vi "re_DataLog Mirror Module.vi"(5 "LuaVIEW reference":T1, 7 "function index":i32) -> (15 "error out":errorcluster)   [LabVIEW 2012]
doc: "Module required by the \"mirroring\" runlevel if mirrored databases have been configured. It assists with the mirroring of a remote logging database. It is reentrant so that it can be instantiated multiple times, once for each database being mirrored."
uses:
  luaview/typedefs/t_LuaVIEW Reference.ctl
  typedefs/clusters/t_DataLog Tag Config.ctl
  typedefs/t_DataLog Temporal Types.ctl
  typedefs/t_DataLog Value Types.ctl
  typedefs/t_DataLog Numerical Format.ctl
  typedefs/t_DataLog Logging Algorithms.ctl
  typedefs/t_DataLog Mirror State Methods.ctl
  clientsrv/served/ClientSrv Server Access_srv.ctl
  clientsrv/typedefs/t_ClientSrv Server Access Methods.ctl
  clientsrv/typedefs/t_ClientSrv Access Levels.ctl
  served/DataLog Mirror_srv.ctl
  served/DataLog Database Infos_srv.ctl
  typedefs/t_DataLog Tag Info List Methods.ctl
  typedefs/t_DataLog Databases Methods.ctl
  luaview/subvis/private/LuaVIEW Pull (flat data).vi
  luaview/subvis/private/LuaVIEW Pull (refnum).vi
  luaview/subvis/private/LuaVIEW Pull (string).vi
  luaview/subvis/private/LuaVIEW Push (string).vi
  luaview/subvis/private/re_LuaVIEW Push (flat data).vi
  luaview/subvis/private/LuaVIEW Push (I32).vi
  luaview/subvis/private/LuaVIEW Pull (I32).vi
  luaview/subvis/private/LuaVIEW Push (boolean).vi
  luaview/subvis/private/LuaVIEW Push (number).vi
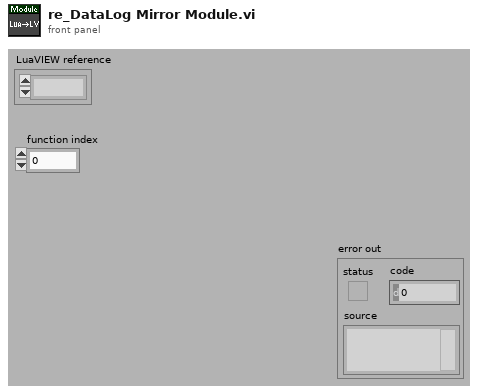
[diagram p1: front panel]
types:
  T1 = typedef "t_LuaVIEW Reference.ctl" = refnum<k1>
  T2 = typedef "t_DataLog Tag Config.ctl" = cluster{"name":string, "unit":string, "temporal":T3, "value":T4, "index":i32, "capacity":i32, "is meta?":bool, "mincapacity":i32, "deadband":dbl, "limit delay":dbl, "format":T5, "precision":u8, "undefine":bool, "update":bool, "update period":u16, "expression":string, "description":string, "logging algorithm":T6, "logging parameters":dbl[]}
  T3 = typedef "t_DataLog Temporal Types.ctl" = enum16{"set&hold", "sample", "event"}
  T4 = typedef "t_DataLog Value Types.ctl" = enum16{"number", "string"}
  T5 = typedef "t_DataLog Numerical Format.ctl" = enum8{"fractional", "exponential", "engineering"}
  T6 = typedef "t_DataLog Logging Algorithms.ctl" = enum16{"nothing", "changes", "everything", "every Nth", "time threshold", "value threshold + prior", "t or v threshold", "t or v threshold + prior"}
  T7 = enum32{"initialize", "str:server=connect()", "num:changecount,tab:taglist=get_list(num:changecount)", "create_empty(tab:config)", "bool:mirrored=mirror_config(tab:remote_config)", "bool:mirrored=mirror_subsets()", "num:mirrored_values=mirror_tag(str:tag)", "str:name=localdb()", "str:name=remotedb()", "disconnect()"}
  T8 = typedef "t_DataLog Mirror State Methods.ctl" = enum16{"add db", "check db", "set", "get", "unset", "clear"}
  T9 = typedef "ClientSrv Server Access_srv.ctl" = refnum<vi>
  T10 = typedef "DataLog Database Infos_srv.ctl" = refnum<vi>
  T11 = typedef "DataLog Mirror_srv.ctl" = refnum<vi>
  T12 = typedef "t_ClientSrv Access Levels.ctl" = enum16{"observer", "operator", "local"}
  T13 = typedef "t_ClientSrv Server Access Methods.ctl" = enum16{"validate access", "test access", "release access", "get name"}
  T14 = typedef "t_DataLog Tag Info List Methods.ctl" = enum16{"initialize", "create", "create empty", "rename", "delete", "test tag", "get", "get by name", "get default", "get list", "get path", "get subsets", "set subsets", "set config", "set capacity", "#tags", "go live", "set unlocked", "set mirrored"}
  T15 = typedef "t_DataLog Databases Methods.ctl" = enum16{"initialize", "get ref", "get names", "cleanup"}
  T16 = cluster{"localdb":string, "remotedb":string, "machine":string, "port":u32, "password":string}
  T17 = enum32{"invalid app kind", "Development System", "Run Time System", "Student Edition", "Embedded LabVIEW", "Evaluation", "Custom"}
  T18 = typedef "t_DataLog Database Info Pane.ctl" = refnum<vi>
  T19 = typedef "et_DataLog Meta Tag Specifier.ctl" = enum32{"warn_lo", "warn_hi", "A_lo", "A_hi", "B_lo", "B_hi", "C_lo", "C_hi", "D_lo", "D_hi", "E_lo", "E_hi", "F_lo", "F_hi", "G_lo", "G_hi", "H_lo", "H_hi", "I_lo", "I_hi", "J_lo", "J_hi", "K_lo", "K_hi", "L_lo", "L_hi", "M_lo", "M_hi", "N_lo", "N_hi", "min", "max", "not a meta"}
  T20 = typedef "t_DataLog Tag Subset.ctl" = cluster{"name":string, "tags":string[]}
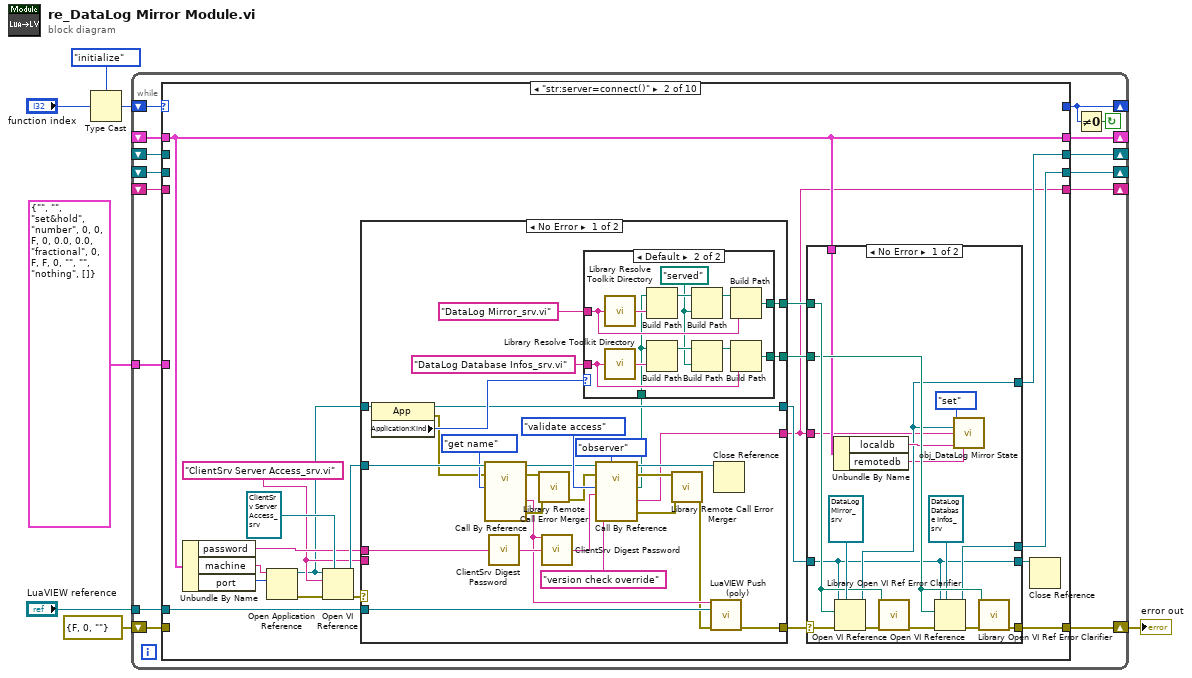
[diagram p0: block diagram]
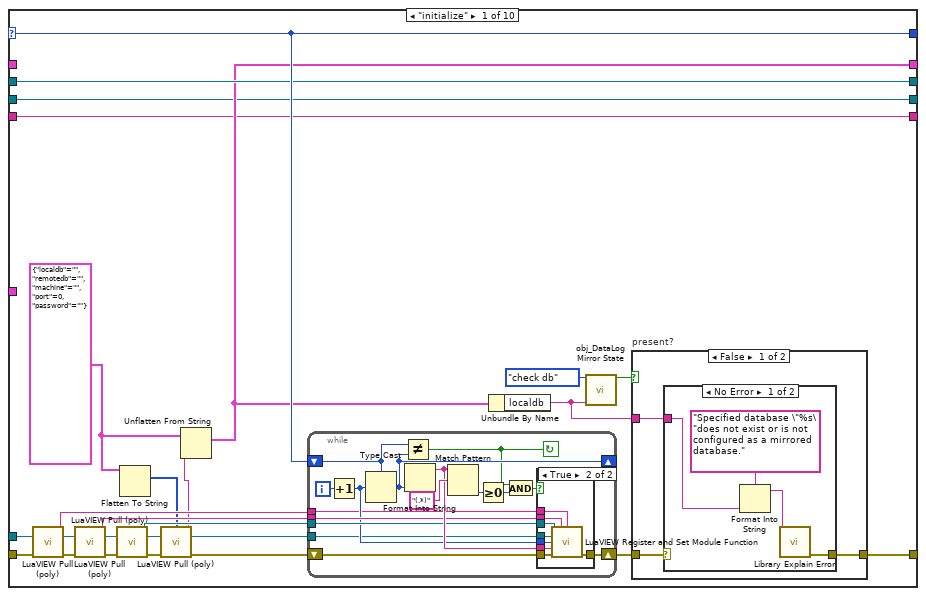
[diagram p2: hidden frame]
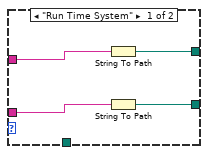
[diagram p7: hidden frame]
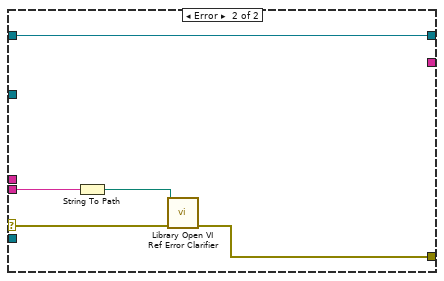
[diagram p8: hidden frame]
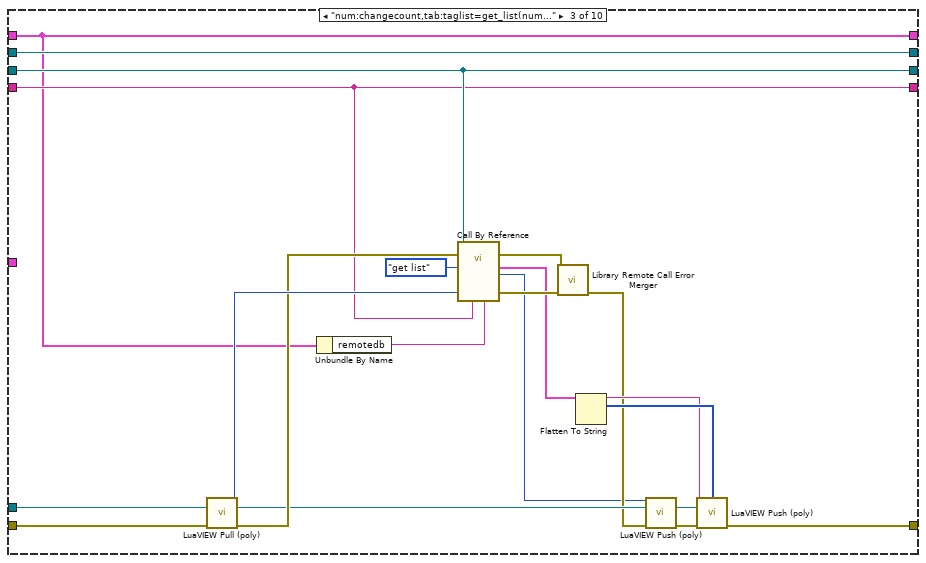
[diagram p9: hidden frame]
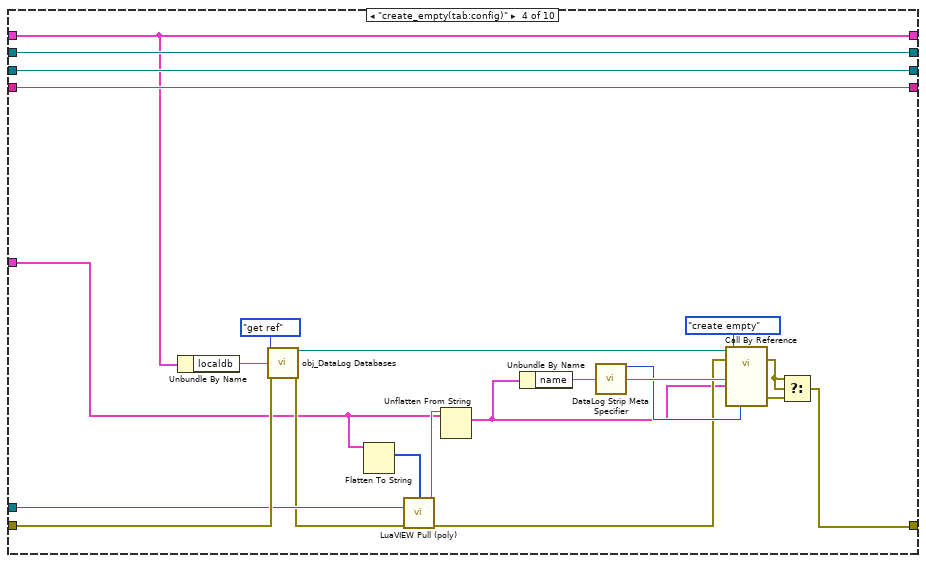
[diagram p10: hidden frame]
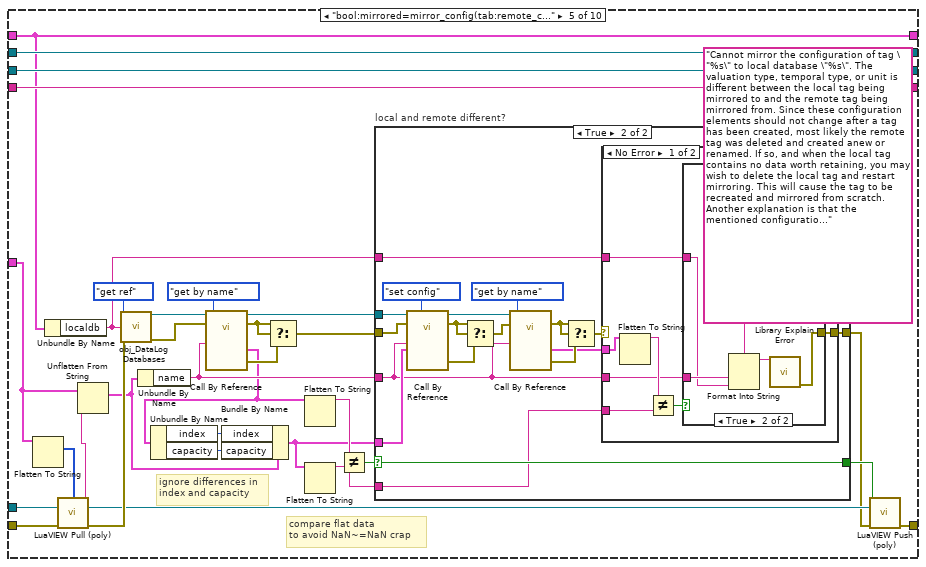
[diagram p11: hidden frame]
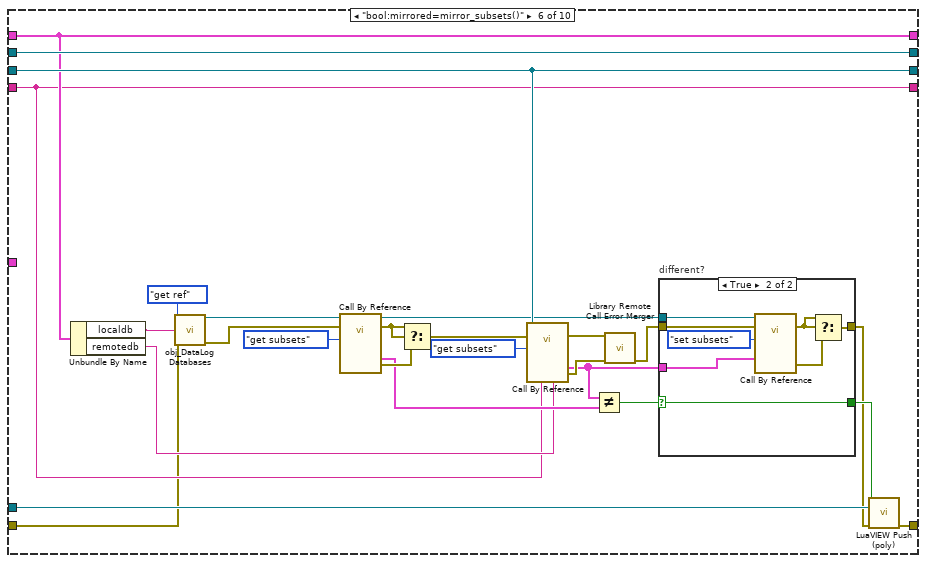
[diagram p15: hidden frame]
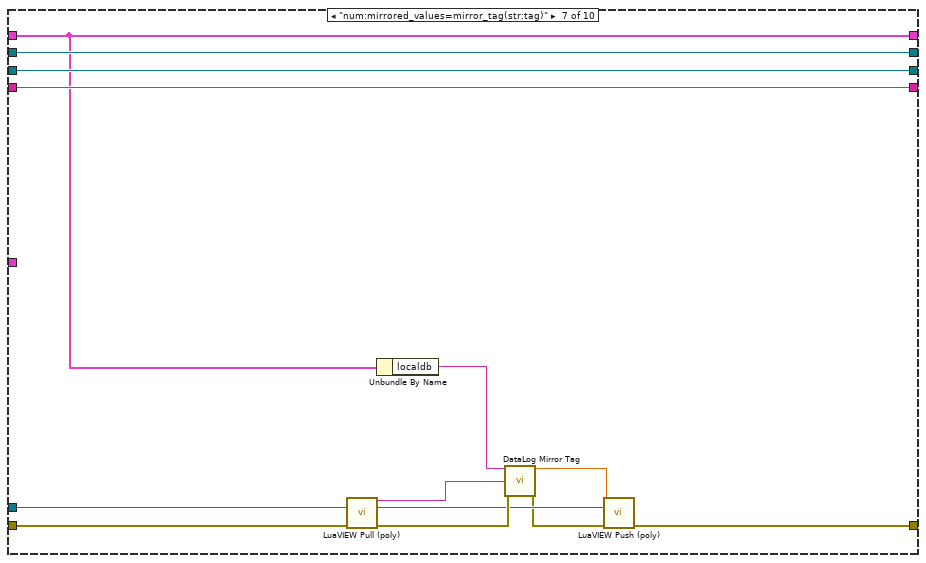
[diagram p17: hidden frame]
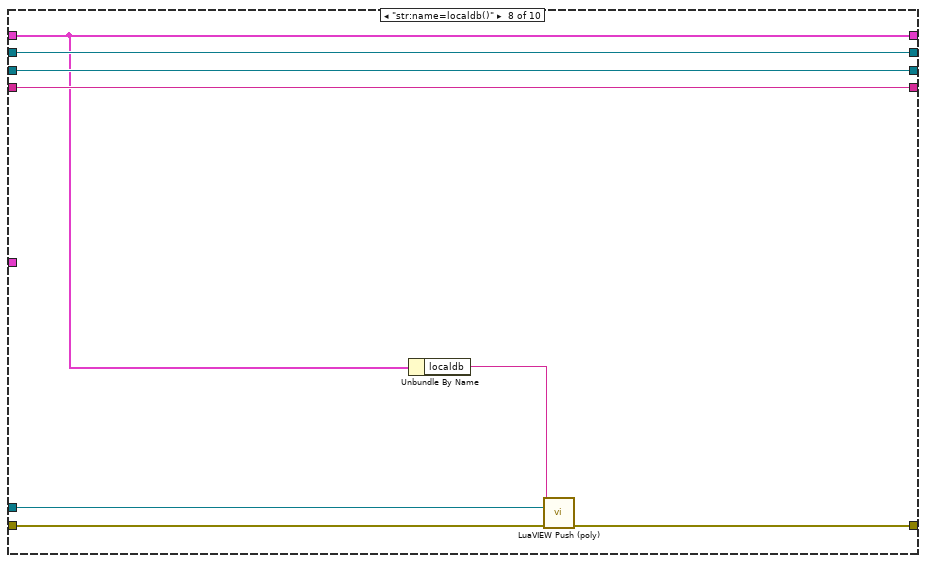
[diagram p18: hidden frame]
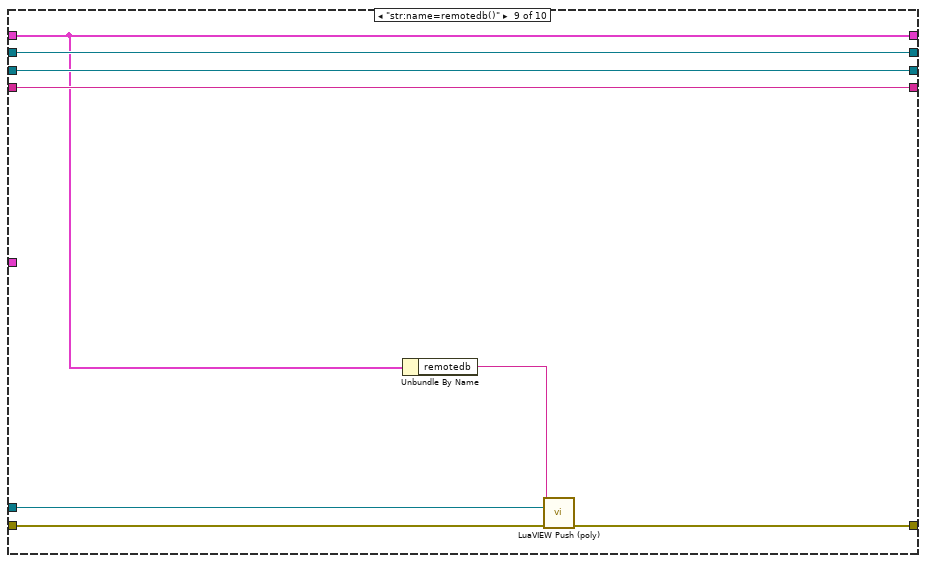
[diagram p19: hidden frame]
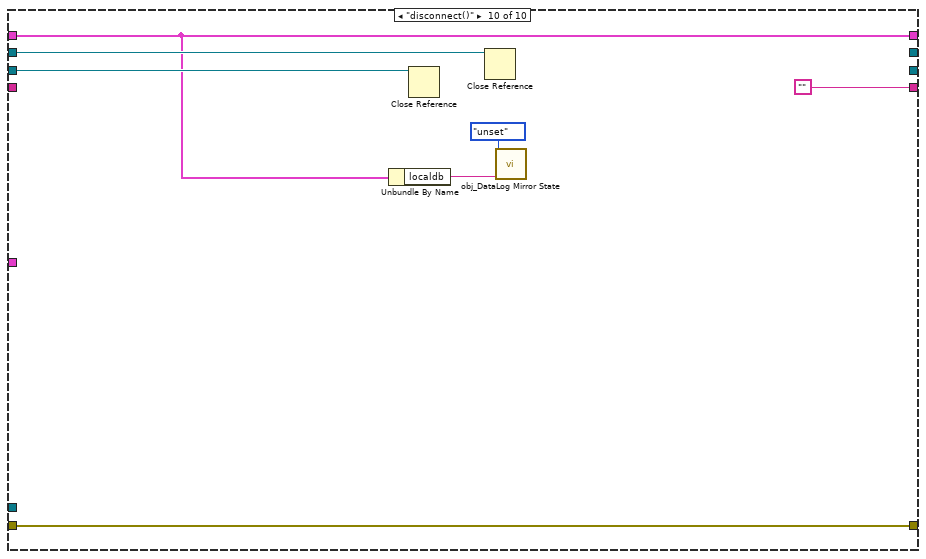
[diagram p20: hidden frame]
diagram:
  n1 = Type Cast(type=T7."initialize" ("cases"), x="function index") -> (*(type *) &x=w6:T7)
  n2 = while {
    shift-right: [w18] -> _
    shift-left: w6 -> [w22]
    shift-right: [w21] -> w7
    shift-left: errorcluster {"status"=FALSE, "code"=0, "source"=""} ("error out") -> [w20]
    tunnel: "LuaVIEW reference" -> [w19]
    shift-right: [w16] -> _
    shift-left: _ -> [w15]
    shift-right: [w14] -> _
    shift-left: _ -> [w13]
    shift-right: [w12] -> _
    shift-left: _ -> [w11]
    shift-right: [w10] -> _
    shift-left: _ -> [w9]
    tunnel: T2 {"name"="", "unit"="", "temporal"=enum."set&hold", "value"=enum."number", "index"=0, "capacity"=0, "is meta?"=FALSE, "mincapacity"=0, "deadband"=0.0, "limit delay"=0.0, "format"=enum."fractional", "precision"=0, "undefine"=FALSE, "update"=FALSE, "update period"=0, "expression"="", "description"="", "logging algorithm"=enum."nothing", "logging parameters"=[]} ("tag config") -> [w8]
    stop <- w17 continue-if-true
    n3 = case shown="\"str:server=connect()\"" w22 {
      selector: w22 -> [w39 _ _ _ _ _ _ _ _ _]
      tunnel: [w39 _ _ _ _ _ _ _ _ _] -> w18
      tunnel: w19 -> [w41 w95 w188 w197 w240 w305 w321 w331 w339 _]
      tunnel: [w27 w93 w183 w203 w226 w304 w317 w330 w338 w351] -> w21
      tunnel: w20 -> [w40 _ w189 w198 w241 w281 w324 w332 w340 w351]
      tunnel: [w31 w85 w173 w202 w243 w298 w325 w333 w341 w347] -> w16
      tunnel: w15 -> [_ w85 w173 w202 w243 w298 w325 w333 w341 w347]
      tunnel: [w32 w86 w192 w214 w246 w303 w328 w336 w344 _] -> w14
      tunnel: w13 -> [w32 _ w192 w214 w246 w303 w328 w336 w344 w350]
      tunnel: [w25 w84 w191 w213 w245 w302 w327 w335 w343 _] -> w12
      tunnel: w11 -> [w25 _ w191 w213 w245 w302 w327 w335 w343 w349]
      tunnel: [w24 w83 w174 w212 w244 w285 w326 w334 w342 ""] -> w10
      tunnel: w9 -> [w24 _ w174 w212 w244 w285 w326 w334 w342 _]
      tunnel: w8 -> [_ _ _ w193 w239 _ _ _ _ _]
      frame "initialize" {
        w23 = T16 {"localdb"="", "remotedb"="", "machine"="", "port"=0, "password"=""} ("server access config out")
        n4 = call-poly "LuaVIEW Pull (poly).vi"("LuaVIEW reference in"=w41, "error in (no error)"=w40) -> ("string"=w44:string, "LuaVIEW reference out"=w46:T1, "error out"=w45:errorcluster)  [unwired: 11 in]
        n5 = call-poly "LuaVIEW Pull (poly).vi"("LuaVIEW reference in"=w46, "error in (no error)"=w45) -> ("string"=w48:string, "LuaVIEW reference out"=w42:T1, "error out"=w43:errorcluster)  [unwired: 11 in]
        n6 = call-poly "LuaVIEW Pull (poly).vi"("LuaVIEW reference in"=w42, "error in (no error)"=w43) -> ("refnum"=w47:refnum<vi>, "LuaVIEW reference out"=w35:T1, "error out"=w36:errorcluster)  [unwired: 11 in]
        n7 = Flatten To String(anything=w23) -> (type string=w38:i16[])  [unwired: 3 in, 2 out]
        n8 = call-poly "LuaVIEW Pull (poly).vi"("type descriptor"=w38, "LuaVIEW reference in"=w35, "error in (no error)"=w36) -> ("flat data"=w37:string, "LuaVIEW reference out"=w34:T1, "error out"=w33:errorcluster)  [unwired: 10 in]
        n9 = Unflatten From String(type=w23, binary string=w37) -> (value=w31:T16)  [unwired: 3 in, 2 out]
        n10 = while {
          tunnel: w44 -> [w62]
          shift-right: [w70] -> w28
          shift-left: w33 -> [w71]
          shift-right: [w66] -> _
          shift-left: w39 -> [w67]
          tunnel: w48 -> [w64]
          tunnel: w47 -> [w65]
          tunnel: w34 -> [w58]
          i -> [w69]
          stop <- w59 continue-if-true
          n11 = Increment(x=w69) -> (x+1=w63:i32)
          n12 = Type Cast(type=w67, x=w63) -> (*(type *) &x=w66:T7)
          n13 = Not Equal?(x=w67, y=w66) -> (x != y?=w59:bool)
          n14 = Format Into String(w66) -> (resulting string=w68:string)  [unwired: 3 in, 1 out]
          n15 = Match Pattern(string=w68, regular expression="(.*)") -> (offset past match=w72:i32)  [unwired: 1 in, 3 out]
          n16 = Greater Or Equal To 0?(x=w72) -> (x >= 0?=w61:bool)
          n17 = And(x=w59, y=w61) -> (x .and. y?=w60:bool)
          n18 = case shown="True" w60 {
            tunnel: w62 -> [_ w76]
            tunnel: w58 -> [_ w80]
            tunnel: w63 -> [_ w81]
            tunnel: w68 -> [_ w78]
            tunnel: [w74 w82] -> w70
            tunnel: w71 -> [w74 w79]
            tunnel: w64 -> [_ w77]
            tunnel: w65 -> [_ w75]
            frame False {
            }
            frame True {
              n19 = call "LuaVIEW Register and Set Module Function.vi"("module refnum"=w75, "export table (set as global)"=w77, "table (set as global)"=w76, "LuaVIEW reference in"=w80, "index"=w81, "synopsis"=w78, "error in (no error)"=w79) -> ("error out"=w82:errorcluster)  [unwired: 7 in, 1 out]
            }
          }
        }
        n20 = Unbundle By Name(w31) -> ("localdb"=w26:string)
        n21 = call "obj_DataLog Mirror State.vi"("method"=t_DataLog_Mirror_State_Methods."check db", "local db"=w26) -> ("present?"=w29:bool)  [unwired: 8 in, 5 out]
        n22 = case "present?" shown="False" w29 {
          tunnel: w28 -> [w51 w57]
          tunnel: [w50 w57] -> w27
          tunnel: w26 -> [w49 _]
          frame False {
            n23 = case shown="No Error" w51 {
              selector: w51 -> [_ w56]
              tunnel: [w55 w56] -> w50
              tunnel: w49 -> [w54 _]
              frame No Error {
                n24 = Format Into String(format string="Specified database \"%s\"does not exist or is not configured as a mirrored database.", w54) -> (resulting string=w53:string)  [unwired: 2 in, 1 out]
                n25 = call "Library Explain Error.vi"("explanation prefix (none)"=w53) -> ("explained error"=w55:errorcluster)  [unwired: 14 in]
              }
              frame Error {
              }
            }
          }
          frame True {
          }
        }
      }
      frame "str:server=connect()" {
        w91 = "ClientSrv Server Access_srv.vi"
        n26 = Unbundle By Name(w85) -> ("password"=w96:string, "machine"=w102:string, "port"=w101:u32)
        n27 = Open Application Reference(10:w101, 11:w102) -> (0:w99:errorcluster, 3:w89:refnum<vi>)  [unwired: 2 in]
        n28 = Open VI Reference(type specifier VI Refnum (for type only)=T9 refnum, application reference (local)=w89, vi path=w91, error in (no error)=w99) -> (vi reference=w97:T9, error out=w98:errorcluster)  [unwired: 2 in]
        n29 = case shown="No Error" w98 {
          selector: w98 -> [_ w171]
          tunnel: w97 -> [w150 _]
          tunnel: [w141 _] -> w83
          tunnel: w96 -> [w137 _]
          tunnel: w91 -> [_ w170]
          tunnel: w95 -> [w133 _]
          tunnel: [w132 w168] -> w94
          tunnel: [w128 w167] -> w90
          tunnel: w89 -> [w131 w167]
          tunnel: [w125 _] -> w87
          tunnel: [w124 _] -> w88
          frame No Error {
            n30 = property class="App"(reference=w131) -> (reference out=w128:refnum<vi>, error out=w123:errorcluster, "Application:Kind"=w129:T17)  [unwired: 1 in]
            n31 = call-by-ref "?"(reference=w150, error in=w123, "method"=t_ClientSrv_Server_Access_Methods."get name") -> (reference out=w143:T9, error out=w148:errorcluster, "certificate/name out"=w134:string, 15:"error out"=w147:errorcluster)  [unwired: 12 in, 1 out]
            n32 = call "ClientSrv Digest Password.vi"("password"=w137) -> ("SHA-1 digest"=w136:string)  [unwired: 14 in]
            n33 = call "Library Remote Call Error Merger.vi"("call by reference node error"=w148, "called VI error (no error)"=w147) -> ("error out"=w140:errorcluster)  [unwired: 13 in]
            n34 = call "ClientSrv Digest Password.vi"("server name (none)"=w134, "password"=w136) -> ("SHA-1 digest"=w138:string)  [unwired: 13 in]
            n35 = call-by-ref "?"(reference=w143, error in=w140, "method"=t_ClientSrv_Server_Access_Methods."validate access", "access level"=t_ClientSrv_Access_Levels."observer", "digest"=w138, "client version"="version check override" ("y")) -> (reference out=w142:T9, error out=w146:errorcluster, "server toolkit path"=w122:path, "certificate/name out"=w141:string, 15:"error out"=w144:errorcluster)  [unwired: 9 in]
            n36 = case shown="Default" w129 {
              tunnel: "DataLog Mirror_srv.vi" -> [w154 w158]
              tunnel: "DataLog Database Infos_srv.vi" -> [w152 w157]
              tunnel: [w151 w160] -> w125
              tunnel: [w153 w159] -> w124
              tunnel: w122 -> [_ w155]
              frame "Run Time System" {
                n37 = String To Path(string=w154) -> (path=w153:path)
                n38 = String To Path(string=w152) -> (path=w151:path)
              }
              frame Default {
                w156 = path "served" ("name or relative path")
                n39 = call "Library Resolve Toolkit Directory.vi"("VI name"=w158) -> ("toolkit directory"=w166:string)
                n40 = call "Library Resolve Toolkit Directory.vi"("VI name"=w157) -> ("toolkit directory"=w161:string)
                n41 = Build Path(base path=w155, name or relative path=w166) -> (appended path=w165:path)
                n42 = Build Path(base path=w155, name or relative path=w161) -> (appended path=w162:path)
                n43 = Build Path(base path=w165, name or relative path=w156) -> (appended path=w164:path)
                n44 = Build Path(base path=w162, name or relative path=w156) -> (appended path=w163:path)
                n45 = Build Path(base path=w164, name or relative path=w158) -> (appended path=w159:path)
                n46 = Build Path(base path=w163, name or relative path=w157) -> (appended path=w160:path)
              }
            }
            n47 = call "Library Remote Call Error Merger.vi"("call by reference node error"=w146, "called VI error (no error)"=w144) -> ("error out"=w130:errorcluster)  [unwired: 13 in]
            n48 = call-poly "LuaVIEW Push (poly).vi"("string"=w134, "LuaVIEW reference in"=w133, "error in (no error)"=w130) -> ("error out"=w132:errorcluster)  [unwired: 11 in, 1 out]
            n49 = Close Reference(reference=w142) -> ()  [unwired: 1 in, 1 out]
          }
          frame Error {
            n50 = String To Path(string=w170) -> (path=w169:path)
            n51 = call "Library Open VI Ref Error Clarifier.vi"("VI path"=w169, "called VI error (no error)"=w171) -> ("error out"=w168:errorcluster)  [unwired: 13 in]
          }
        }
        n52 = case shown="No Error" w94 {
          selector: w94 -> [w118 w121]
          tunnel: [w114 w121] -> w93
          tunnel: w90 -> [w103 w120]
          tunnel: [w103 w120] -> w92
          tunnel: [w106 _] -> w86
          tunnel: w88 -> [w116 _]
          tunnel: w87 -> [w112 _]
          tunnel: w85 -> [w110 _]
          tunnel: [w107 _] -> w84
          tunnel: w83 -> [w105 _]
          frame No Error {
            n53 = Unbundle By Name(w110) -> ("localdb"=w109:string, "remotedb"=w104:string)
            n54 = Open VI Reference(type specifier VI Refnum (for type only)=T11 refnum, application reference (local)=w103, vi path=w116, error in (no error)=w118) -> (vi reference=w106:T11, error out=w117:errorcluster)  [unwired: 2 in]
            n55 = call "Library Open VI Ref Error Clarifier.vi"("VI path"=w116, "called VI error (no error)"=w117) -> ("error out"=w113:errorcluster)  [unwired: 13 in]
            n56 = Open VI Reference(type specifier VI Refnum (for type only)=T10 refnum, application reference (local)=w103, vi path=w112, error in (no error)=w113) -> (vi reference=w107:T10, error out=w115:errorcluster)  [unwired: 2 in]
            n57 = call "obj_DataLog Mirror State.vi"("method"=t_DataLog_Mirror_State_Methods."set", "mirror in"=w106, "certificate in"=w105, "local db"=w109, "remote db in"=w104) -> ()  [unwired: 5 in, 6 out]
            n58 = call "Library Open VI Ref Error Clarifier.vi"("VI path"=w112, "called VI error (no error)"=w115) -> ("error out"=w114:errorcluster)  [unwired: 13 in]
          }
          frame Error {
          }
        }
        n59 = Close Reference(reference=w92) -> ()  [unwired: 1 in, 1 out]
      }
      frame "num:changecount,tab:taglist=get_list(num:changecount)" {
        n60 = call-poly "LuaVIEW Pull (poly).vi"("LuaVIEW reference in"=w188, "error in (no error)"=w189) -> ("I32"=w187:i32, "LuaVIEW reference out"=w179:T1, "error out"=w186:errorcluster)  [unwired: 11 in]
        n61 = Unbundle By Name(w173) -> ("remotedb"=w172:string)
        n62 = call-by-ref "?"(reference=w191, error in=w186, "method"=t_DataLog_Tag_Info_List_Methods."get list", "meta specifier (not a meta)"=w187, "certificate in"=w174, "database (current)"=w172) -> (error out=w185:errorcluster, "tag config list"=w182:T2[], "#tags/change#"=w176:i32, 15:"error out"=w184:errorcluster)  [unwired: 6 in, 4 out]
        n63 = call "Library Remote Call Error Merger.vi"("call by reference node error"=w185, "called VI error (no error)"=w184) -> ("error out"=w177:errorcluster)  [unwired: 13 in]
        n64 = Flatten To String(anything=w182) -> (data string=w180:string, type string=w181:i16[])  [unwired: 3 in, 1 out]
        n65 = call-poly "LuaVIEW Push (poly).vi"("I32"=w176, "LuaVIEW reference in"=w179, "error in (no error)"=w177) -> ("LuaVIEW reference out"=w178:T1, "error out"=w175:errorcluster)  [unwired: 11 in]
        n66 = call-poly "LuaVIEW Push (poly).vi"("flat data"=w180, "type descriptor"=w181, "LuaVIEW reference in"=w178, "error in (no error)"=w175) -> ("error out"=w183:errorcluster)  [unwired: 10 in, 1 out]
      }
      frame "create_empty(tab:config)" {
        n67 = Unbundle By Name(w202) -> ("localdb"=w201:string)
        n68 = call "obj_DataLog Databases.vi"("method"=t_DataLog_Databases_Methods."get ref", "database (current)"=w201, "error in (no error)"=w198) -> ("database ref"=w199:T18, "error out"=w196:errorcluster)  [unwired: 10 in, 1 out]
        n69 = Flatten To String(anything=w193) -> (type string=w210:i16[])  [unwired: 3 in, 2 out]
        n70 = call-poly "LuaVIEW Pull (poly).vi"("type descriptor"=w210, "LuaVIEW reference in"=w197, "error in (no error)"=w196) -> ("flat data"=w209:string, "error out"=w204:errorcluster)  [unwired: 10 in, 1 out]
        n71 = Unflatten From String(type=w193, binary string=w209) -> (value=w195:T2)  [unwired: 3 in, 2 out]
        n72 = Unbundle By Name(w195) -> ("name"=w194:string)
        n73 = call "DataLog Strip Meta Specifier.vi"("tag"=w194) -> ("meta specifier"=w205:T19, "base tag"=w206:string)  [unwired: 13 in]
        n74 = call-by-ref "?"(reference=w199, error in=w204, "method"=t_DataLog_Tag_Info_List_Methods."create empty", "tag or base tag"=w206, "tag config in"=w195, "meta specifier (not a meta)"=w205) -> (error out=w207:errorcluster, 15:"error out"=w208:errorcluster)  [unwired: 5 in, 7 out]
        n75 = Select(t=w207, s=w207, f=w208) -> (s? t:f=w203:errorcluster)
      }
      frame "bool:mirrored=mirror_config(tab:remote_config)" {
        # "ignore differences in\nindex and capacity"
        # "compare flat data\nto avoid NaN~=NaN crap"
        n76 = Flatten To String(anything=w239) -> (type string=w242:i16[])  [unwired: 3 in, 2 out]
        n77 = Unbundle By Name(w243) -> ("localdb"=w221:string)
        n78 = call-poly "LuaVIEW Pull (poly).vi"("type descriptor"=w242, "LuaVIEW reference in"=w240, "error in (no error)"=w241) -> ("flat data"=w223:string, "LuaVIEW reference out"=w227:T1, "error out"=w232:errorcluster)  [unwired: 10 in]
        n79 = Unflatten From String(type=w239, binary string=w223) -> (value=w220:T2)  [unwired: 3 in, 2 out]
        n80 = call "obj_DataLog Databases.vi"("method"=t_DataLog_Databases_Methods."get ref", "database (current)"=w221, "error in (no error)"=w232) -> ("database ref"=w237:T18, "error out"=w236:errorcluster)  [unwired: 10 in, 1 out]
        n81 = Unbundle By Name(w220) -> ("name"=w228:string)
        n82 = call-by-ref "?"(reference=w237, error in=w236, "method"=t_DataLog_Tag_Info_List_Methods."get by name", "tag or base tag"=w228) -> (reference out=w224:T18, error out=w235:errorcluster, "tag config out"=w219:T2, 15:"error out"=w234:errorcluster)  [unwired: 7 in, 5 out]
        n83 = Unbundle By Name(w219) -> ("index"=w218:i32, "capacity"=w217:i32)
        n84 = Bundle By Name(cluster=w220, "index"=w218, "capacity"=w217) -> (w216:T2)
        n85 = Select(t=w235, s=w235, f=w234) -> (s? t:f=w229:errorcluster)
        n86 = Flatten To String(anything=w219) -> (data string=w231:string)  [unwired: 3 in, 2 out]
        n87 = Flatten To String(anything=w216) -> (data string=w215:string)  [unwired: 3 in, 2 out]
        n88 = Not Equal?(x=w231, y=w215) -> (x != y?=w230:bool)
        n89 = case "local and remote different?" shown="True" w230 {
          selector: w230 -> [w247 w262]
          tunnel: w229 -> [w248 w264]
          tunnel: w228 -> [_ w250]
          tunnel: w216 -> [_ w263]
          tunnel: [w247 w262] -> w225
          tunnel: w224 -> [_ w258]
          tunnel: w215 -> [_ w251]
          tunnel: [w248 w253] -> w222
          tunnel: w221 -> [_ w249]
          frame False {
          }
          frame True {
            n90 = call-by-ref "?"(reference=w258, error in=w264, "method"=t_DataLog_Tag_Info_List_Methods."set config", "tag or base tag"=w250, "tag config in"=w263) -> (reference out=w256:T18, error out=w257:errorcluster, 15:"error out"=w265:errorcluster)  [unwired: 6 in, 6 out]
            n91 = Select(t=w257, s=w257, f=w265) -> (s? t:f=w259:errorcluster)
            n92 = call-by-ref "?"(reference=w256, error in=w259, "method"=t_DataLog_Tag_Info_List_Methods."get by name", "tag or base tag"=w250) -> (error out=w261:errorcluster, "tag config out"=w252:T2, 15:"error out"=w260:errorcluster)  [unwired: 7 in, 6 out]
            n93 = Select(t=w261, s=w261, f=w260) -> (s? t:f=w254:errorcluster)
            n94 = case shown="No Error" w254 {
              selector: w254 -> [_ w279]
              tunnel: [w268 w279] -> w253
              tunnel: w252 -> [w273 _]
              tunnel: w251 -> [w271 _]
              tunnel: w250 -> [w269 _]
              tunnel: w249 -> [w267 _]
              frame No Error {
                n95 = Flatten To String(anything=w273) -> (data string=w272:string)  [unwired: 3 in, 2 out]
                n96 = Not Equal?(x=w272, y=w271) -> (x != y?=w270:bool)
                n97 = case shown="True" w270 {
                  tunnel: w269 -> [_ w278]
                  tunnel: [_ w276] -> w268
                  tunnel: w267 -> [_ w274]
                  frame False {
                  }
                  frame True {
                    n98 = Format Into String(format string="Cannot mirror the configuration of tag \"%s\" to local database \"%s\". The valuation type, temporal type, or unit is different between the local tag being mirrored to and the remote tag being mirrored from. Since these configuration elements should not change after a tag has been created, most likely the remote tag was deleted and created anew or renamed. If so, and when the local tag contains no data worth retaining, you may wish to delete the local tag and restart mirroring. This will cause the tag to be recreated and mirrored from scratch. Another explanation is that the mentioned configuration elements of the remote tag were intentionally modified by directly editing its on-disk configuration file. If so, do the same for the local tag. Beware that the databases runlevel may not be active while doing so.", w278, w274) -> (resulting string=w277:string)  [unwired: 2 in, 1 out]
                    n99 = call "Library Explain Error.vi"("explanation prefix (none)"=w277) -> ("explained error"=w276:errorcluster)  [unwired: 14 in]
                  }
                }
              }
              frame Error {
              }
            }
          }
        }
        n100 = call-poly "LuaVIEW Push (poly).vi"("boolean"=w225, "LuaVIEW reference in"=w227, "error in (no error)"=w222) -> ("error out"=w226:errorcluster)  [unwired: 11 in, 1 out]
      }
      frame "bool:mirrored=mirror_subsets()" {
        n101 = Unbundle By Name(w298) -> ("localdb"=w300:string, "remotedb"=w286:string)
        n102 = call "obj_DataLog Databases.vi"("method"=t_DataLog_Databases_Methods."get ref", "database (current)"=w300, "error in (no error)"=w281) -> ("database ref"=w297:T18, "error out"=w296:errorcluster)  [unwired: 10 in, 1 out]
        n103 = call-by-ref "?"(reference=w297, error in=w296, "method"=t_DataLog_Tag_Info_List_Methods."get subsets") -> (reference out=w289:T18, error out=w295:errorcluster, "subsets out"=w288:T20[], 15:"error out"=w294:errorcluster)  [unwired: 8 in, 5 out]
        n104 = Select(t=w295, s=w295, f=w294) -> (s? t:f=w293:errorcluster)
        n105 = call-by-ref "?"(reference=w302, error in=w293, "method"=t_DataLog_Tag_Info_List_Methods."get subsets", "certificate in"=w285, "database (current)"=w286) -> (error out=w291:errorcluster, "subsets out"=w284:T20[], 15:"error out"=w290:errorcluster)  [unwired: 7 in, 5 out]
        n106 = Not Equal?(x=w284, y=w288) -> (x != y?=w283:bool)
        n107 = call "Library Remote Call Error Merger.vi"("call by reference node error"=w291, "called VI error (no error)"=w290) -> ("error out"=w287:errorcluster)  [unwired: 13 in]
        n108 = case "different?" shown="True" w283 {
          selector: w283 -> [w307 w313]
          tunnel: w289 -> [_ w315]
          tunnel: w287 -> [w306 w314]
          tunnel: w284 -> [_ w309]
          tunnel: [w307 w313] -> w282
          tunnel: [w306 w308] -> w280
          frame False {
          }
          frame True {
            n109 = call-by-ref "?"(reference=w315, error in=w314, "method"=t_DataLog_Tag_Info_List_Methods."set subsets", "subsets in"=w309) -> (error out=w311:errorcluster, 15:"error out"=w310:errorcluster)  [unwired: 7 in, 7 out]
            n110 = Select(t=w311, s=w311, f=w310) -> (s? t:f=w308:errorcluster)
          }
        }
        n111 = call-poly "LuaVIEW Push (poly).vi"("boolean"=w282, "LuaVIEW reference in"=w305, "error in (no error)"=w280) -> ("error out"=w304:errorcluster)  [unwired: 11 in, 1 out]
      }
      frame "num:mirrored_values=mirror_tag(str:tag)" {
        n112 = call-poly "LuaVIEW Pull (poly).vi"("LuaVIEW reference in"=w321, "error in (no error)"=w324) -> ("string"=w320:string, "LuaVIEW reference out"=w319:T1, "error out"=w322:errorcluster)  [unwired: 11 in]
        n113 = Unbundle By Name(w325) -> ("localdb"=w323:string)
        n114 = call "DataLog Mirror Tag.vi"("local db"=w323, "tag"=w320, "error in (no error)"=w322) -> ("mirrored values"=w316:dbl, "error out"=w318:errorcluster)  [unwired: 11 in]
        n115 = call-poly "LuaVIEW Push (poly).vi"("number"=w316, "LuaVIEW reference in"=w319, "error in (no error)"=w318) -> ("error out"=w317:errorcluster)  [unwired: 11 in, 1 out]
      }
      frame "str:name=localdb()" {
        n116 = Unbundle By Name(w333) -> ("localdb"=w329:string)
        n117 = call-poly "LuaVIEW Push (poly).vi"("string"=w329, "LuaVIEW reference in"=w331, "error in (no error)"=w332) -> ("error out"=w330:errorcluster)  [unwired: 11 in, 1 out]
      }
      frame "str:name=remotedb()" {
        n118 = Unbundle By Name(w341) -> ("remotedb"=w337:string)
        n119 = call-poly "LuaVIEW Push (poly).vi"("string"=w337, "LuaVIEW reference in"=w339, "error in (no error)"=w340) -> ("error out"=w338:errorcluster)  [unwired: 11 in, 1 out]
      }
      frame "disconnect()" {
        n120 = Unbundle By Name(w347) -> ("localdb"=w345:string)
        n121 = Close Reference(reference=w349) -> ()  [unwired: 1 in, 1 out]
        n122 = Close Reference(reference=w350) -> ()  [unwired: 1 in, 1 out]
        n123 = call "obj_DataLog Mirror State.vi"("method"=t_DataLog_Mirror_State_Methods."unset", "local db"=w345) -> ()  [unwired: 8 in, 6 out]
      }
    }
    n124 = Not Equal To 0?(x=w18) -> (x != 0?=w17:bool)
  }
  "error out" <- w7
